vi "Latch_withEnable_2.vi"(3 "Enable":bool, 5 "D":dbl) -> (1 "Q":dbl)   [LabVIEW 2020]
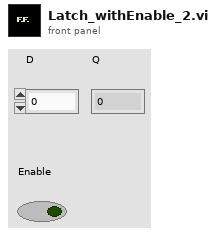
[diagram p1: front panel]
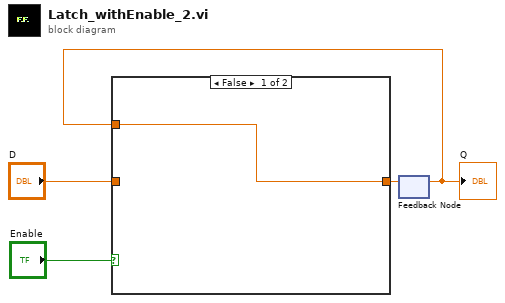
[diagram p0: block diagram]
diagram:
  n1 = feedback #1() -> (w1:dbl)  [unwired: 1 in]
  "Q" <- w1
  n2 = case shown="False" "Enable" {
    tunnel: "D" -> [_ w6]
    tunnel: [w5 w6] -> w2
    tunnel: w1 -> [w5 _]
    frame False {
    }
    frame True {
    }
  }
  n3 = feedback-in #1(w2) -> ()
